vi "Inspect.vi"(10 "Msg in":refnum<class "Msg.lvclass">, 11 "jettl Actor in":refnum<class "jettl Actor.lvclass">) -> (2 "Msg out":refnum<class "Msg.lvclass">, 3 "jettl Actor out":refnum<class "jettl Actor.lvclass">)   [LabVIEW 2021, in "jettl.lvlib" / "Temporary Actor.lvlib" / "jettl Actor.lvclass"]
uses:
  jettl Actor.lvclass
  Msg/Msg.lvclass
  jettl Actor.lvclass/jettl Actor.ctl
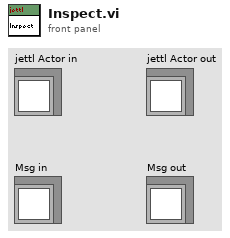
[diagram p1: front panel]
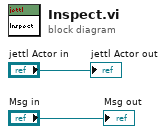
[diagram p0: block diagram]
diagram:
  "jettl Actor out" <- "jettl Actor in"
  "Msg out" <- "Msg in"
